vi "启动整机测试 (子VI).vi"   [LabVIEW 2016]
uses:
  PLC/PLC.lvlib
types:
  T1 = enum32{"Bad", "Idle", "Run top level", "Running"}
  T2 = cluster{"多参数":bool, "CODMn":bool, "总磷总氮":bool, "氨氮":bool, "CODcr":bool}
  T3 = cluster{"启动测量模式":cluster{"测量模式":enum16{"水样测量", "标样核查", "零点核查", "跨度核查", "加标回收", "平行样", "校零", "校标"}}, "确定按钮":bool}
  T4 = cluster{"CODCr":cluster{"启动测量模式":cluster{"测量模式":enum16{"水样测量", "标样核查", "零点核查", "跨度核查", "加标回收", "平行样", "校零", "校标"}}, "确定按钮":bool}, "参数启用":cluster{"多参数":bool, "CODMn":bool, "总磷总氮":bool, "氨氮":bool, "CODcr":bool}}
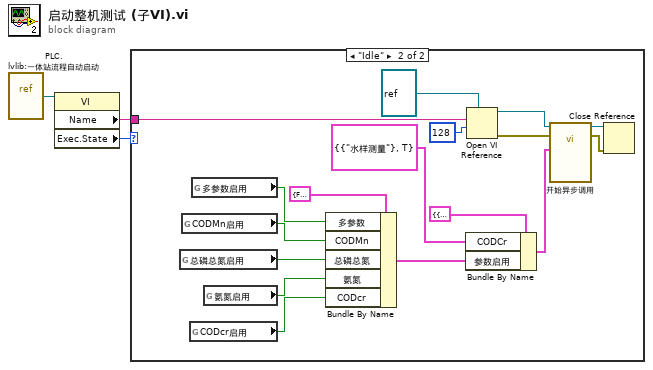
[diagram p0: block diagram]
diagram:
  n1 = vi-ref "PLC.lvlib:一体站流程自动启动.vi"() -> (w2:refnum<vi>)
  n2 = property class="VI"(reference=w2) -> ("Name"=w3:string, "Exec.State"=w1:T1)  [unwired: 1 in, 2 out]
  n3 = case shown="\"Idle\"" w1 {
    tunnel: w3 -> [_ w14]
    frame "Bad", Default {
    }
    frame "Idle" {
      n4 = global read "系统设置全局变量.vi" "总磷总氮启用"() -> (w6:bool)
      n5 = global read "系统设置全局变量.vi" "CODMn启用"() -> (w7:bool)
      n6 = global read "系统设置全局变量.vi" "CODcr启用"() -> (w4:bool)
      n7 = global read "系统设置全局变量.vi" "多参数启用"() -> (w8:bool)
      n8 = global read "系统设置全局变量.vi" "氨氮启用"() -> (w5:bool)
      n9 = Bundle By Name(cluster=T2 {"多参数"=FALSE, "CODMn"=FALSE, "总磷总氮"=FALSE, "氨氮"=FALSE, "CODcr"=FALSE} ("参数启用"), "多参数"=w8, "CODMn"=w7, "总磷总氮"=w6, "氨氮"=w5, "CODcr"=w4) -> (w9:T2)
      n10 = Bundle By Name(cluster=T4 {"CODCr"={"启动测量模式"={"测量模式"=enum."水样测量"}, "确定按钮"=FALSE}, "参数启用"={"多参数"=FALSE, "CODMn"=FALSE, "总磷总氮"=FALSE, "氨氮"=FALSE, "CODcr"=FALSE}} ("参数"), "CODCr"=T3 {"启动测量模式"={"测量模式"=enum."水样测量"}, "确定按钮"=TRUE}, "参数启用"=w9) -> (w12:T4)
      n11 = Open VI Reference(type specifier VI Refnum (for type only)=refnum<vi> refnum, vi path=w14, options=128 ("选项")) -> (vi reference=w16:refnum<vi>, error out=w19:errorcluster)  [unwired: 3 in]
      n12 = call-by-ref "开始异步调用"(reference=w16, error in=w19, "参数"=w12) -> (reference out=w18:refnum<vi>, error out=w20:errorcluster)  [unwired: 11 in]
      n13 = Close Reference(reference=w18, error in (no error)=w20) -> ()  [unwired: 1 out]
    }
  }
